vi "Read BM Messages.vi"(0 "Bus Config Info":T1, 11 "error in (no error)":errorcluster) -> (4 "VP BM Messages Read":T3[](array[typedef]) {"Data Word array" format="%x"}, 8 "Data Available":bool, 15 "error out":errorcluster)   [LabVIEW 2013]
uses:
  RT Controls/VP_BM Message.ctl
  RT Controls/AIT 1553 - Board Config Info.ctl
  RT Controls/AIT 1553 - Hardware Type.ctl
  <instrlib>/AIT 1553/AIT 1553.lvlib
  AIT 664 Custom Device.lvlib
  <userlib>/MIL-STD-1553/Owl1553.lvlib
  <vilib>/NI Veristand/Custom Device Tools/Custom Device Utility Library/Custom Device Utility Library.lvlib
panel:
  out "BM Read Exec Time":u32
  out "words read out":i32
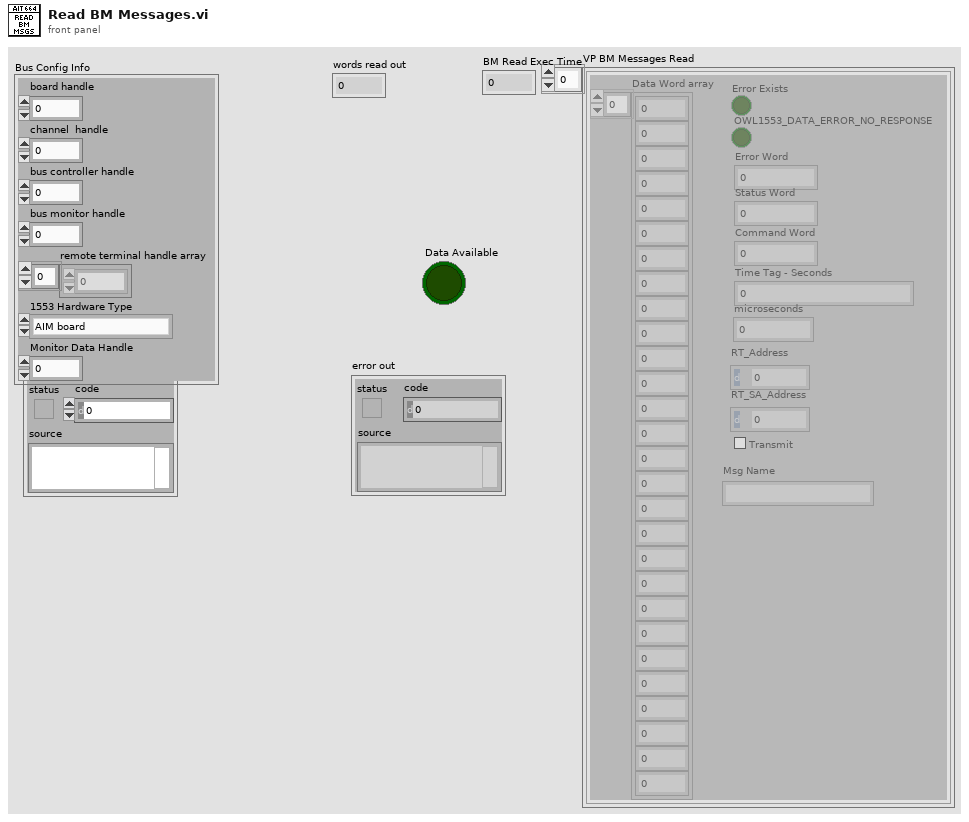
[diagram p1: front panel]
types:
  T1 = typedef "AIT 664 Custom Device.lvlib/AIT 1553 - Board Config Info.ctl" = cluster{"board handle":u32, "channel  handle":u32, "bus controller handle":u32, "bus monitor handle":u32, "remote terminal handle array":u32[], "1553 Hardware Type":T2, "Monitor Data Handle":u32}
  T2 = typedef "AIT 664 Custom Device.lvlib/AIT 1553 - Hardware Type.ctl" = enum16{"AIM board", "AIT Board"}
  T3 = typedef "AIT 664 Custom Device.lvlib/VP_BM Message.ctl" = cluster{"Data Word array":u16[], "Error Exists":bool, "OWL1553_DATA_ERROR_NO_RESPONSE":bool, "Error Word":u32, "Status Word":u16, "Command Word":u16, "Time Tag - Seconds":u32, "microseconds":u32, "RT_Address":u8, "RT_SA_Address":u8, "Transmit":bool, "Msg Name":string}
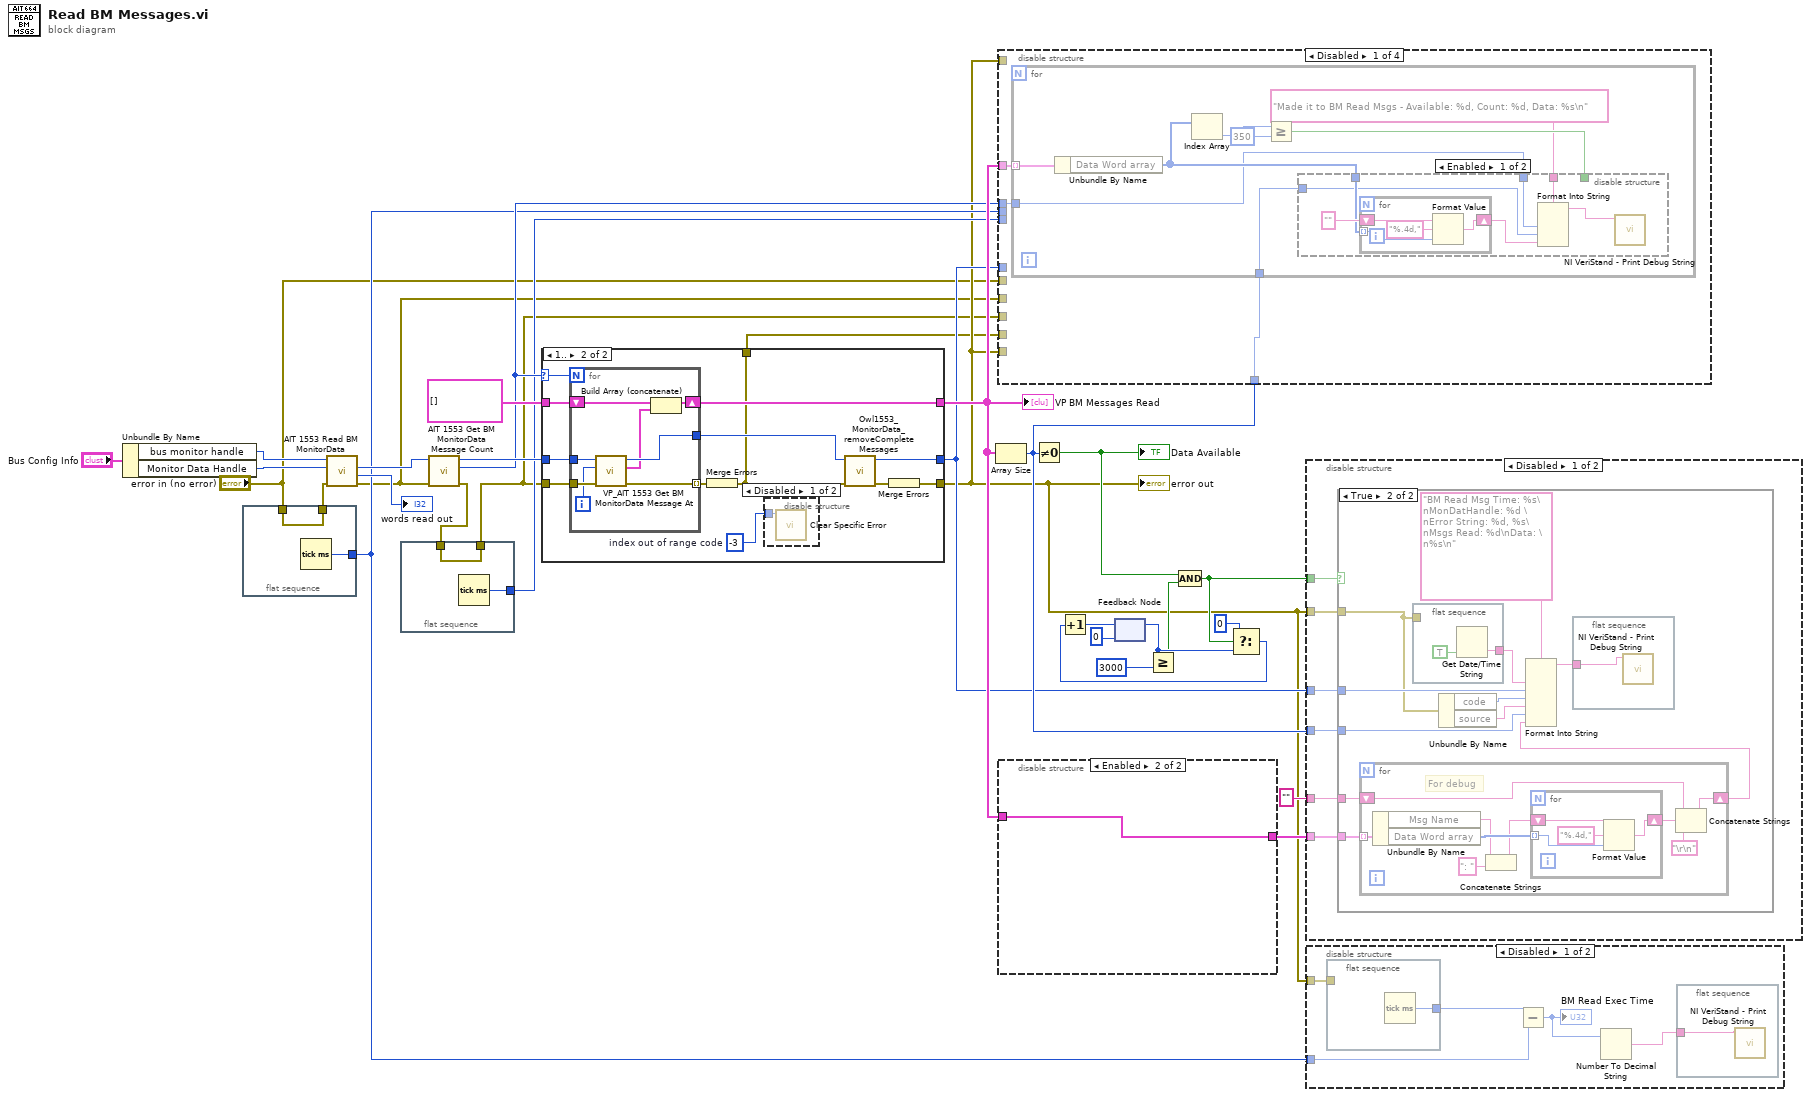
[diagram p0: block diagram]
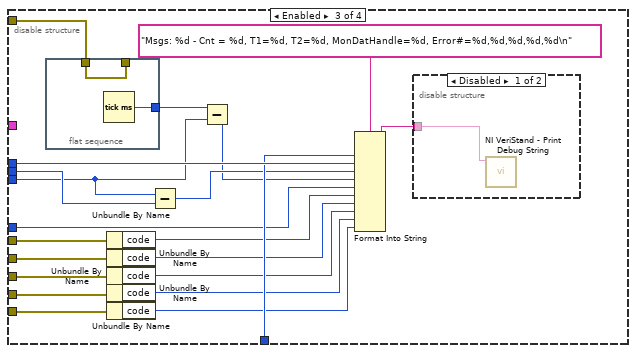
[diagram p4: hidden frame]
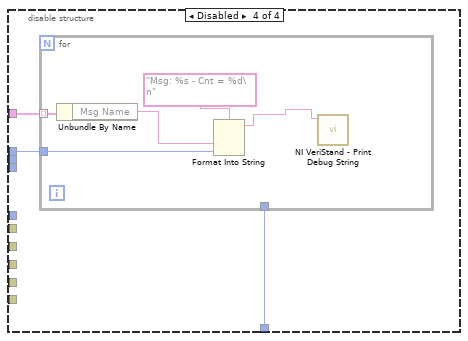
[diagram p6: hidden frame]
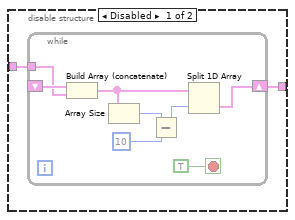
[diagram p10: hidden frame]
diagram:
  n1 = Unbundle By Name("Bus Config Info") -> ("bus monitor handle"=w5:u32, "Monitor Data Handle"=w26:u32)
  n2 = flat-sequence {
    tunnel: "error in (no error)" -> [w33]
    tunnel: [w33] -> w15
    tunnel: [w32] -> w9
    frame #0 {
      n3 = Tick Count (ms)() -> (millisecond timer value=w32:u32)
    }
  }
  n4 = call <instrlib>:"AIT 1553 Read BM MonitorData.vi"("error in"=w15, "monitor data handle in"=w26, "bus monitor handle in"=w5) -> ("error out"=w3:errorcluster, "words read out"=→"words read out":i32, "monitor data handle out"=w30:u64)  [unwired: 5 in, 1 out]
  n5 = flat-sequence {
    tunnel: w10 -> [w35]
    tunnel: [w35] -> w2
    tunnel: [w34] -> w8
    frame #0 {
      n6 = Tick Count (ms)() -> (millisecond timer value=w34:u32)
    }
  }
  n7 = call <instrlib>:"AIT 1553 Get BM MonitorData Message Count.vi"("error in"=w3, "monitor data handle in"=w30) -> ("error out"=w10:errorcluster, "message count out"=w12:u32, "monitor data handle out"=w29:u64)  [unwired: 7 in]
  n8 = case shown="1.." w12 {
    selector: w12 -> [_ w45]
    tunnel: w2 -> [w36 w50]
    tunnel: w29 -> [w37 w48]
    tunnel: T3[] [] -> [w38 w47]
    tunnel: [w38 w46] -> w14
    tunnel: [w36 w42] -> w6
    tunnel: [w37 w44] -> w7
    tunnel: [_ w40] -> w1
    frame 0, Default {
    }
    frame 1.. {
      w39 = -3  # index out of range code
      n9 = for {
        N: w45 -> [_]
        tunnel: w50 -> [w59]
        tunnel: [w58] -> w49 mode=indexing
        tunnel: w48 -> [w57]
        shift-right: [w54] -> w46
        shift-left: w47 -> [w55]
        tunnel: [w53] -> w43
        i -> [w56]
        n10 = call "VP_AIT 1553 Get BM MonitorData Message At.vi"("error in"=w59, "message index in"=w56, "monitor data handle in"=w57) -> ("error out"=w58:errorcluster, "VP BM Message"=w52:T3[], "monitor data handle out"=w53:u32)  [unwired: 5 in]
        n11 = Build Array (concatenate)(w55, w52) -> (w54:T3[])
      }
      n12 = Merge Errors(w49) -> (w40:errorcluster)
      n13 = disable-structure shown="Disabled" {
        disable-tunnel: w39 -> [w51 _]
        frame Disabled {
          n14 = call "Clear Specific Error.vi"("code"=w51) -> ()  [unwired: 9 in, 2 out]
        }
        frame Enabled {
        }
      }
      n15 = call <userlib>:"Owl1553_MonitorData_removeCompleteMessages.vi"("error in (no error)"=w40, "monitor data handle"=w43) -> ("error out"=w41:errorcluster, "monitor data handle"=w44:u64)  [unwired: 8 in]
      n16 = Merge Errors(w41) -> (w42:errorcluster)
    }
  }
  "error out" <- w6
  "VP BM Messages Read" <- w14
  n17 = Array Size(array=w14) -> (size(s)=w13:i32)
  n18 = disable-structure shown="Disabled" {
    disable-tunnel: w14 -> [w62 _ _ w108]
    disable-tunnel: w13 -> [w61 _ w99 w107]
    disable-tunnel: w12 -> [w60 _ w102 w106]
    disable-tunnel: w9 -> [_ _ w97 _]
    disable-tunnel: w8 -> [_ _ w94 _]
    disable-tunnel: w6 -> [_ _ w98 _]
    disable-tunnel: w7 -> [_ _ w92 _]
    disable-tunnel: w6 -> [_ _ w88 _]
    disable-tunnel: "error in (no error)" -> [_ _ w91 _]
    disable-tunnel: w3 -> [_ _ w90 _]
    disable-tunnel: w2 -> [_ _ w89 _]
    disable-tunnel: w1 -> [_ _ w87 _]
    frame Disabled {
      n19 = for {
        tunnel: w62 -> [w67] mode=indexing
        tunnel: w61 -> [w64]
        tunnel: w60 -> [w63]
        n20 = Unbundle By Name(w67) -> ("Data Word array"=w70:u16[])
        n21 = Index Array(array=w70) -> (element=w69:u16)  [unwired: 1 in]
        n22 = Greater Or Equal?(x=w69, y=u16 350) -> (x >= y?=w66:bool)
        n23 = disable-structure shown="Enabled" {
          disable-tunnel: "Made it to BM Read Msgs - Available: %d, Count: %d, Data: %s\n" ("format string") -> [w76 _]
          disable-tunnel: w70 -> [w74 _]
          disable-tunnel: w66 -> [_ _]
          disable-tunnel: w64 -> [w73 _]
          disable-tunnel: w63 -> [w72 _]
          frame Enabled {
            n24 = for {
              tunnel: w74 -> [w78] mode=indexing
              shift-right: [w79] -> w75
              shift-left: "" ("format string") -> [w80]
              n25 = Format Value(string ("")=w80, format string="%.4d,", value (0)=w78) -> (output string=w79:string)
            }
            n26 = Format Into String(format string=w76, w72, w73, w75) -> (resulting string=w71:string)  [unwired: 2 in, 1 out]
            n27 = call <vilib>:"NI VeriStand - Print Debug String.vi"("Message"=w71) -> ()  [unwired: 10 in, 1 out]
          }
          frame Disabled {
          }
        }
      }
    }
    frame Disabled {
    }
    frame Enabled {
      n28 = flat-sequence {
        tunnel: w98 -> [w105]
        tunnel: [w105] -> _
        tunnel: [w104] -> w95
        frame #0 {
          n29 = Tick Count (ms)() -> (millisecond timer value=w104:u32)
        }
      }
      n30 = Unbundle By Name(w91) -> ("code"=w86:i32)
      n31 = Unbundle By Name(w90) -> ("code"=w85:i32)
      n32 = Unbundle By Name(w89) -> ("code"=w84:i32)
      n33 = Unbundle By Name(w87) -> ("code"=w83:i32)
      n34 = Unbundle By Name(w88) -> ("code"=w82:i32)
      n35 = Subtract(x=w94, y=w97) -> (x-y=w96:u32)
      n36 = Subtract(x=w95, y=w94) -> (x-y=w93:u32)
      n37 = Format Into String(format string="Msgs: %d - Cnt = %d, T1=%d, T2=%d, MonDatHandle=%d, Error#=%d,%d,%d,%d,%d\n", w99, w102, w96, w93, w92, w86, w85, w84, w83, w82) -> (resulting string=w101:string)  [unwired: 2 in, 1 out]
      n38 = disable-structure shown="Disabled" {
        disable-tunnel: w101 -> [w103 _]
        frame Disabled {
          n39 = call <vilib>:"NI VeriStand - Print Debug String.vi"("Message"=w103) -> ()  [unwired: 10 in, 1 out]
        }
        frame Enabled {
        }
      }
    }
    frame Disabled {
      n40 = for {
        tunnel: w108 -> [w112] mode=indexing
        tunnel: w107 -> [_]
        tunnel: w106 -> [w110]
        n41 = Unbundle By Name(w112) -> ("Msg Name"=w111:string)
        n42 = Format Into String(format string="Msg: %s - Cnt = %d\n", w111, w110) -> (resulting string=w109:string)  [unwired: 2 in, 1 out]
        n43 = call <vilib>:"NI VeriStand - Print Debug String.vi"("Message"=w109) -> ()  [unwired: 10 in, 1 out]
      }
    }
  }
  n44 = disable-structure shown="Enabled" {
    disable-tunnel: w14 -> [w115 w124]
    disable-tunnel: [w114 w124] -> w17
    frame Disabled {
      n45 = while {
        shift-right: [w120] -> w114
        shift-left: _ -> [w122]
        tunnel: w115 -> [w121]
        stop <- TRUE stop-if-true
        n46 = Build Array (concatenate)(w122, w121) -> (w119:T3[])
        n47 = Array Size(array=w119) -> (size(s)=w118:i32)
        n48 = Subtract(x=w118, y=10 ("index")) -> (x-y=w116:i32)
        n49 = Split 1D Array(array=w119, index=w116) -> (second subarray=w120:T3[])  [unwired: 1 out]
      }
    }
    frame Enabled {
    }
  }
  n50 = Not Equal To 0?(x=w13) -> (x != 0?=w21:bool)
  "Data Available" <- w21
  n51 = feedback #1(0) -> (w19:i32)
  n52 = Greater Or Equal?(x=w19, y=3000) -> (x >= y?=w11:bool)
  n53 = Compound Arithmetic op=AND(w21, w11) -> (w16:bool)
  n54 = Select(t=0, s=w16, f=w19) -> (s? t:f=w18:i32)
  n55 = Increment(x=w18) -> (x+1=w24:i32)
  n56 = feedback-in #1(w24) -> ()
  n57 = disable-structure shown="Disabled" {
    disable-tunnel: w13 -> [w130 _]
    disable-tunnel: w6 -> [w129 _]
    disable-tunnel: w7 -> [w128 _]
    disable-tunnel: "" ("format string") -> [w127 _]
    disable-tunnel: w17 -> [w126 _]
    disable-tunnel: w16 -> [w125 _]
    frame Disabled {
      n58 = case shown="True" w125 {
        tunnel: w128 -> [_ w136]
        tunnel: w130 -> [_ w135]
        tunnel: w129 -> [_ w134]
        tunnel: w126 -> [_ w133]
        tunnel: w127 -> [_ w132]
        frame False {
        }
        frame True {
          n59 = for {
            tunnel: w133 -> [w150] mode=indexing
            shift-right: [w146] -> w131
            shift-left: w132 -> [w145]
            # "For debug"
            n60 = Unbundle By Name(w150) -> ("Msg Name"=w144:string, "Data Word array"=w149:u16[])
            n61 = Concatenate Strings(w144, ": " ("string")) -> (w142:string)
            n62 = for {
              tunnel: w149 -> [w151] mode=indexing
              shift-right: [w152] -> w148
              shift-left: w142 -> [w153]
              n63 = Format Value(string ("")=w153, format string="%.4d,", value (0)=w151) -> (output string=w152:string)
            }
            n64 = Concatenate Strings(w145, w148, "\r\n") -> (w146:string)
          }
          n65 = flat-sequence {
            tunnel: [w156] -> w137
            tunnel: w134 -> [_]
            frame #0 {
              n66 = Get Date/Time String(want seconds? (F)=TRUE) -> (time string=w156:string)  [unwired: 2 in, 1 out]
            }
          }
          n67 = Unbundle By Name(w134) -> ("code"=w140:i32, "source"=w141:string)
          n68 = Format Into String(format string="BM Read Msg Time: %s\nMonDatHandle: %d \nError String: %d, %s\nMsgs Read: %d\nData: \n%s\n", w137, w136, w140, w141, w135, w131) -> (resulting string=w139:string)  [unwired: 2 in, 1 out]
          n69 = flat-sequence {
            tunnel: w139 -> [w157]
            frame #0 {
              n70 = call <vilib>:"NI VeriStand - Print Debug String.vi"("Message"=w157) -> ()  [unwired: 10 in, 1 out]
            }
          }
        }
      }
    }
    frame Enabled {
    }
  }
  n71 = disable-structure shown="Disabled" {
    disable-tunnel: w6 -> [w162 _]
    disable-tunnel: w9 -> [w160 _]
    frame Disabled {
      n72 = flat-sequence {
        tunnel: w162 -> [_]
        tunnel: [w164] -> w161
        frame #0 {
          n73 = Tick Count (ms)() -> (millisecond timer value=w164:u32)
        }
      }
      n74 = Subtract(x=w161, y=w160) -> (x-y=w159:u32)
      "BM Read Exec Time" <- w159
      n75 = Number To Decimal String(number=w159) -> (decimal integer string=w158:string)  [unwired: 1 in]
      n76 = flat-sequence {
        tunnel: w158 -> [w163]
        frame #0 {
          n77 = call <vilib>:"NI VeriStand - Print Debug String.vi"("Message"=w163) -> ()  [unwired: 10 in, 1 out]
        }
      }
    }
    frame Enabled {
    }
  }
